vi "Open.vi"(8 "error in (no error)":errorcluster, 10 "Send \"Connect client\"":bool, 11 "RP Communicator in":refnum<class "RP Communicator VISA.lvclass">) -> (0 "error out":errorcluster, 3 "RP Communicator out":refnum<class "RP Communicator VISA.lvclass">)   [LabVIEW 2015, in "RP Communicator VISA.lvclass"]
uses:
  RP Communicator VISA.lvclass
  <vilib>/Instr/_visa.llb/VISA Open Access Mode.ctl
  RP Communicator VISA.lvclass/RP Communicator VISA.ctl
  RP Command.ctl
  RP Write Command VISA.vi
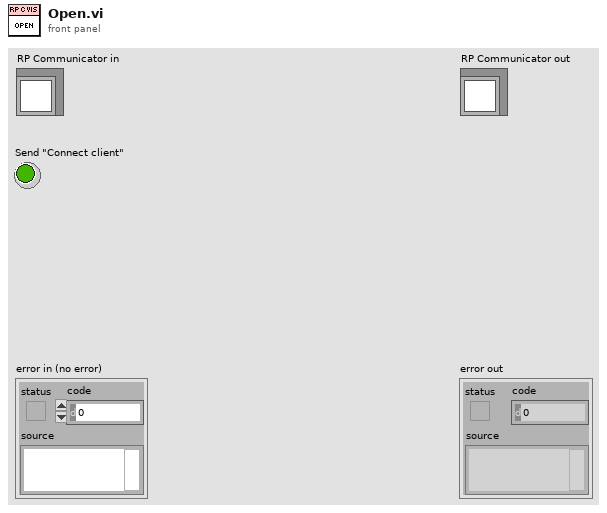
[diagram p1: front panel]
types:
  T1 = typedef "RP Command.ctl" = enum16{"Reset", "Read IDN", "Stop server", "Get status", "Get temperature", "Connect client", "Arm", "Software trigger", "Get whole buffer", "Get chunk", "System call", "Get config", "Set config", "Recieve data", "Play pattern", "Transmit data"}
  T2 = typedef "VISA Open Access Mode.ctl" = u32
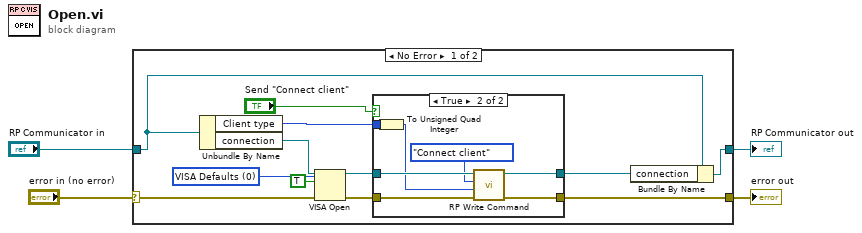
[diagram p0: block diagram]
diagram:
  n1 = case shown="No Error" "error in (no error)" {
    selector: "error in (no error)" -> [w16 w27]
    tunnel: [w9 w27] -> w3
    tunnel: [w11 w26] -> w1
    tunnel: "RP Communicator in" -> [w12 w26]
    frame No Error {
      w5 = T2 0 items=["VISA Defaults"=0, "Exclusive Lock"=1, "Load Configured Settings"=4] ("Access Mode")
      n2 = Unbundle By Name(w12) -> ("Client type"=w13:enum16{"Control", "Reciever", "Transmitter"}, "connection"=w7:refnum<visa-resource-name>)
      n3 = VISA Open(duplicate session (F)=TRUE, access mode=w5, error in (no error)=w16, VISA resource name=w7) -> (VISA resource name=w14:refnum<visa-resource-name>, error out=w15:errorcluster)  [unwired: 1 in]
      n4 = case shown="True" "Send \"Connect client\"" {
        tunnel: w15 -> [w17 w25]
        tunnel: w14 -> [w18 w24]
        tunnel: w13 -> [_ w22]
        tunnel: [w18 w20] -> w10
        tunnel: [w17 w19] -> w9
        frame False {
        }
        frame True {
          n5 = To Unsigned Quad Integer(1:w22) -> (0:w21:u64)
          n6 = call-poly "RP Write Command.vi"("Error In"=w25, "Command payload"=w21, "Command number"=RP_Command."Connect client", "VISA resource"=w24) -> ("Error Out"=w19:errorcluster, "VISA resource out"=w20:refnum<visa-resource-name>)  [unwired: 5 in, 1 out]
        }
      }
      n7 = Bundle By Name(cluster=w12, "connection"=w10) -> (w11:refnum<class "RP Communicator VISA.lvclass">)
    }
    frame Error {
    }
  }
  "error out" <- w3
  "RP Communicator out" <- w1
